vi "Destroy Events.vi"(8 "error in (no error)":errorcluster, 11 "Motor Controller in":refnum<class "Motor Controller.lvclass">) -> (0 "error out":errorcluster, 3 "Motor Controller out":refnum<class "Motor Controller.lvclass">)   [LabVIEW 2022 SP3, in "Motor Controller.lvclass"]
uses:
  Motor Controller.lvclass
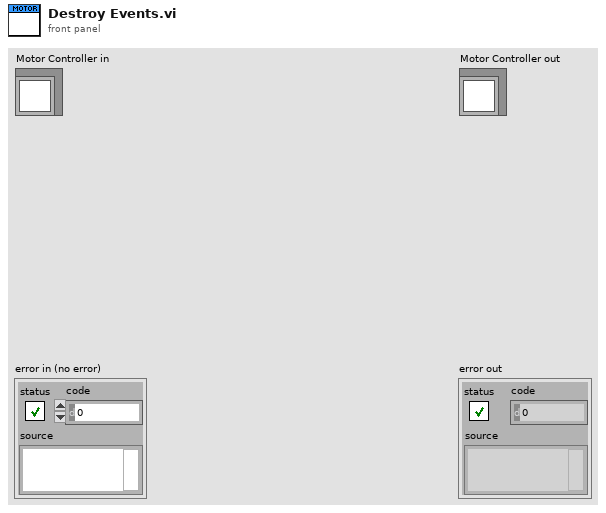
[diagram p1: front panel]
types:
  T1 = typedef "Motor Controller.lvclass/UserEvents.ctl" = cluster{"API Incoming Event":refnum<user-event>, "API Executed Event":refnum<user-event>, "API Return Event":refnum<user-event>, "Status Changed Event":refnum<user-event>, "StopEvent":refnum<user-event>}
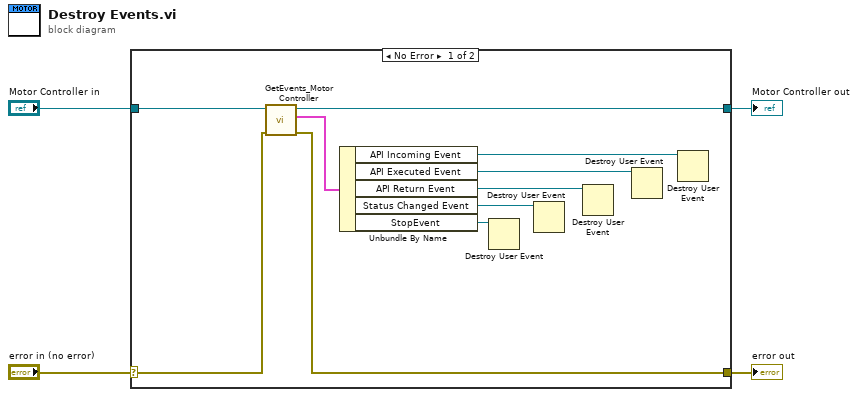
[diagram p0: block diagram]
diagram:
  n1 = case shown="No Error" "error in (no error)" {
    selector: "error in (no error)" -> [w6 w16]
    tunnel: [w5 w16] -> w3
    tunnel: [w14 w15] -> w1
    tunnel: "Motor Controller in" -> [w13 w15]
    frame No Error {
      n2 = call-dynamic "GetEvents_Motor Controller.vi"("error in (no error)"=w6, "TopLevel in"=w13) -> ("error out"=w5:errorcluster, "UserEvents"=w9:T1, "TopLevel out"=w14:refnum<class "Motor Controller.lvclass">)  [unwired: 7 in]
      n3 = Unbundle By Name(w9) -> ("API Incoming Event"=w10:refnum<user-event>, "API Executed Event"=w11:refnum<user-event>, "API Return Event"=w12:refnum<user-event>, "Status Changed Event"=w8:refnum<user-event>, "StopEvent"=w7:refnum<user-event>)
      n4 = Destroy User Event(user event=w7) -> ()  [unwired: 1 in, 1 out]
      n5 = Destroy User Event(user event=w8) -> ()  [unwired: 1 in, 1 out]
      n6 = Destroy User Event(user event=w12) -> ()  [unwired: 1 in, 1 out]
      n7 = Destroy User Event(user event=w11) -> ()  [unwired: 1 in, 1 out]
      n8 = Destroy User Event(user event=w10) -> ()  [unwired: 1 in, 1 out]
    }
    frame Error {
    }
  }
  "error out" <- w3
  "Motor Controller out" <- w1
